vi "Turret_Native_Units_To_Degrees.vi"(1 "Native Units":dbl) -> (0 "Degrees":dbl)   [LabVIEW 2019]
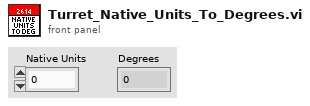
[diagram p1: front panel]
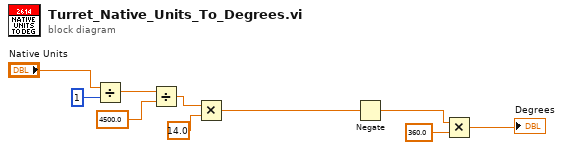
[diagram p0: block diagram]
diagram:
  n1 = Divide(x="Native Units", y=1) -> (x/y=w2:dbl)
  n2 = Divide(x=w2, y=4500.0) -> (x/y=w4:dbl)
  n3 = Multiply(x=w4, y=14.0) -> (x*y=w6:dbl)
  n4 = Negate(x=w6) -> (-x=w10:dbl)
  n5 = Multiply(x=w10, y=360.0) -> (x*y=→"Degrees":dbl)
